vi "Global.vi"() -> ()   [LabVIEW 2015]
panel:
  in  "5190settingsIdx4":dbl[](array[numeric])
  in  "5190settingsIdx3":dbl[](array[numeric])
  in  "5190settingsIdx2":dbl[](array[numeric])
  in  "5190settingsIdx1":dbl[](array[numeric])
  in  "5190settingsIdx0":dbl[](array[numeric])
  in  "5190settingsGlobal":dbl[][](array[numeric])
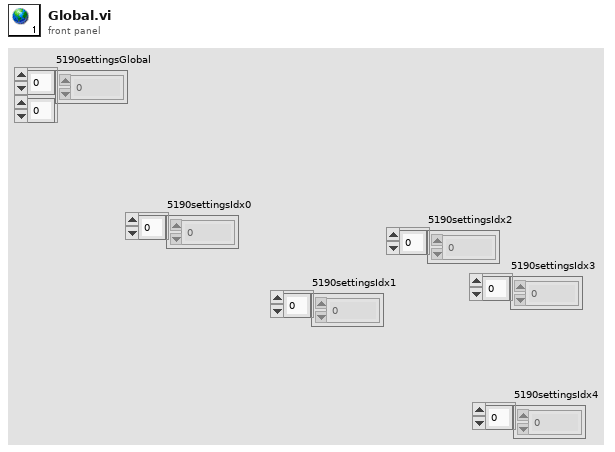
[diagram p1: front panel]
diagram:
